vi "Set Configuration.vi"(8 "error in (no error)":errorcluster, 11 "EST Bidirectional Sensor in":refnum<class "EST Bidirectional Sensor.lvclass">) -> (0 "error out":errorcluster, 3 "EST Bidirectional Sensor out":refnum<class "EST Bidirectional Sensor.lvclass">)   [LabVIEW 2015, in "EST Bidirectional Sensor.lvclass"]
uses:
  EST Bidirectional Sensor.lvclass
  IO Class/Type.ctl
  EST Output/EST Output.lvclass
  IO Class/IO Class.lvclass
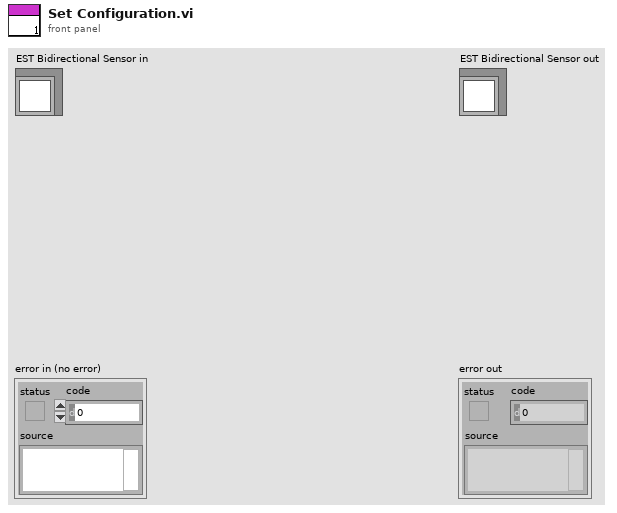
[diagram p1: front panel]
types:
  T1 = typedef "IO Class.lvclass/Type.ctl" = cluster{"Type":string}
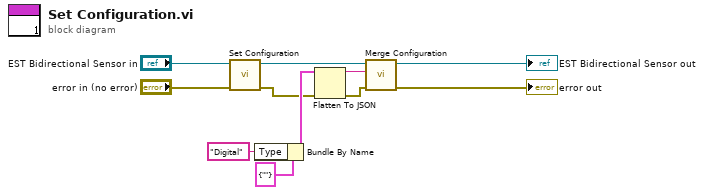
[diagram p0: block diagram]
diagram:
  n1 = call-parent "Set Configuration.vi"("error in (no error)"="error in (no error)", "EST Output in"="EST Bidirectional Sensor in") -> ("error out"=w5:errorcluster, "EST Output out"=w6:refnum<class "EST Bidirectional Sensor.lvclass">)  [unwired: 8 in]
  n2 = Bundle By Name(cluster=T1 {"Type"=""} ("Type"), "Type"="Digital") -> (w10:T1)
  n3 = Flatten To JSON(anything=w10, error in (no error)=w5) -> (JSON string=w8:string, 11:w7:errorcluster)  [unwired: 1 in]
  n4 = call "Merge Configuration.vi"("error in (no error)"=w7, "Additional Configuration"=w8, "IO Class in"=w6) -> ("error out"=→"error out":errorcluster, "IO Class out"=→"EST Bidirectional Sensor out":refnum<class "EST Bidirectional Sensor.lvclass">)  [unwired: 7 in]
